vi "mongo_cursor_init.vi"(9 "ns":string, 10 "conn ptr":u32, 11 "cursor ptr":u32) -> (2 "conn ptr out":u32, 3 "cursor ptr out":u32)   [LabVIEW 2013]
uses:
  mongo-c-driver/libmongoc.so
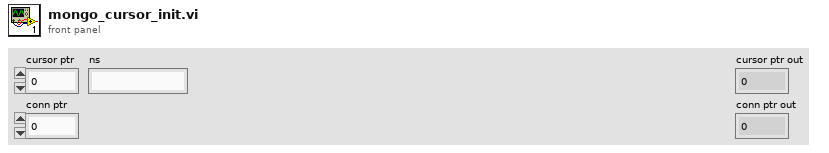
[diagram p1: front panel]
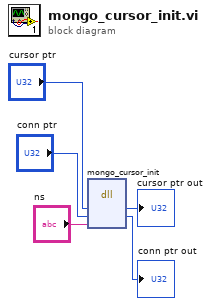
[diagram p0: block diagram]
diagram:
  n1 = dll-call lib="home/scot/dev/git/mongo-c-driver/libmongoc.so" fn="mongo_cursor_init"("cursor ptr"="cursor ptr", "conn ptr"="conn ptr", "ns"="ns") -> ("cursor ptr"=→"cursor ptr out":u32, "conn ptr"=→"conn ptr out":u32)  [unwired: 5 in, 2 out]
